vi "is over thershold.vi"(10 "Avg HR":dbl, 11 "Array":dbl[](array[numeric])) -> (3 "Boolean":bool)   [LabVIEW 2014]
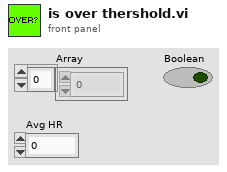
[diagram p1: front panel]
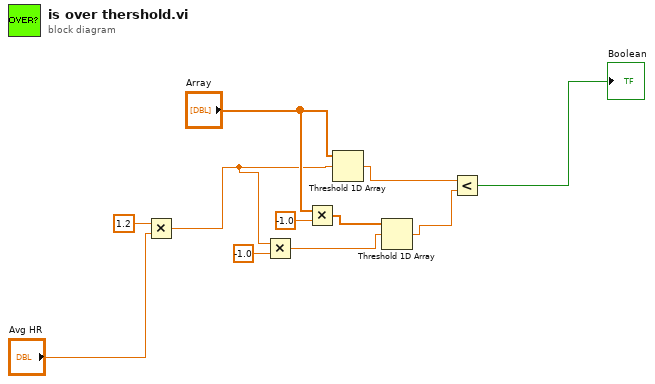
[diagram p0: block diagram]
diagram:
  n1 = Multiply(x=1.2, y="Avg HR") -> (x*y=w1:dbl)
  n2 = Multiply(x=w1, y=-1.0) -> (x*y=w8:dbl)
  n3 = Multiply(x="Array", y=-1.0) -> (x*y=w7:dbl[])
  n4 = Threshold 1D Array(2:w1, 3:"Array") -> (0:w9:dbl)  [unwired: 1 in]
  n5 = Threshold 1D Array(2:w8, 3:w7) -> (0:w10:dbl)  [unwired: 1 in]
  n6 = Less?(x=w9, y=w10) -> (x < y?=→"Boolean":bool)
